vi "GetAbortedStatus.vi"(8 "error in (no error)":errorcluster, 11 "UI_Interaction_Manager in":refnum<class "UI_Interaction_Manager.lvclass">) -> (0 "error out":errorcluster, 2 "Aborted?":bool, 3 "UI_Interaction_Manager out":refnum<class "UI_Interaction_Manager.lvclass">)   [LabVIEW 2011, in "UI_Interaction_Manager.lvclass"]
uses:
  UI_Interaction_Manager.lvclass
  UI_Interaction_Manager.lvclass/UI_Interaction_Manager.ctl
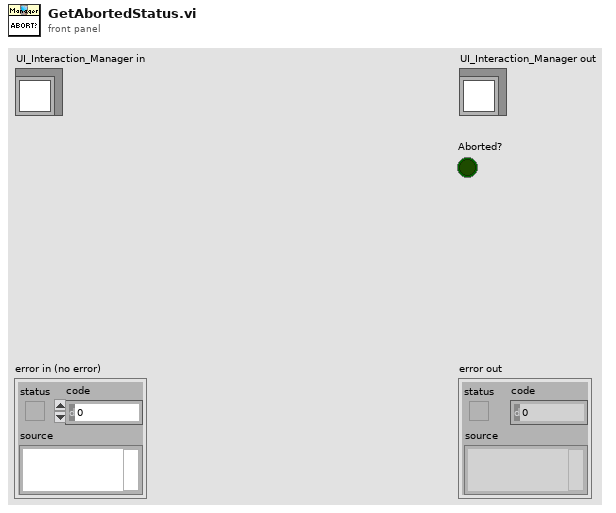
[diagram p1: front panel]
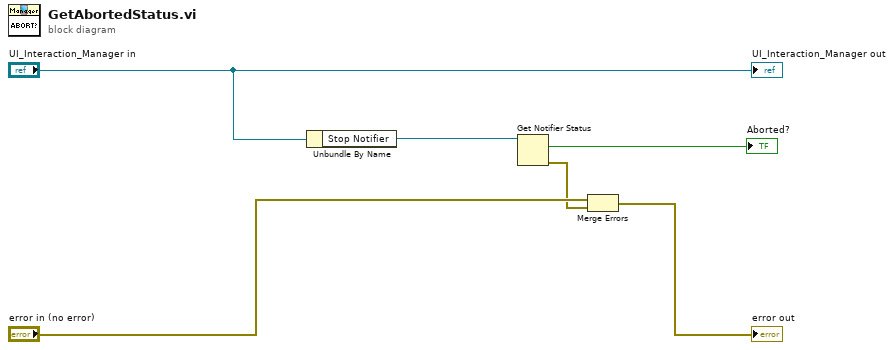
[diagram p0: block diagram]
diagram:
  n1 = Unbundle By Name("UI_Interaction_Manager in") -> ("Stop Notifier"=w4:refnum<notifier>)
  n2 = Get Notifier Status(notifier=w4) -> (current notification=→"Aborted?":bool, error out=w2:errorcluster)  [unwired: 1 in, 3 out]
  n3 = Merge Errors("error in (no error)", w2) -> (→"error out":errorcluster)
  "UI_Interaction_Manager out" <- "UI_Interaction_Manager in"
